vi "Configure Filter.vi"(8 "error in (no error)":errorcluster, 9 "Set Filter (1: On)":i32(ring)=1 items=["Off", "On"], 10 "Select Filter Type (0 : Frequency)":u32(ring) items=["Frequency", "Line"], 11 "VISA resource name":refnum<visa-resource-name>) -> (0 "error out":errorcluster, 3 "VISA resource name out":refnum<visa-resource-name>)   [LabVIEW 2019, in "Yokogawa WT300 Series.lvlib"]
doc: "Configures the frequency or Line filter features."
uses:
  Yokogawa WT300 Series.lvlib
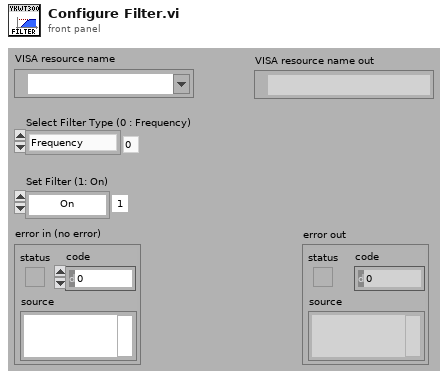
[diagram p1: front panel]
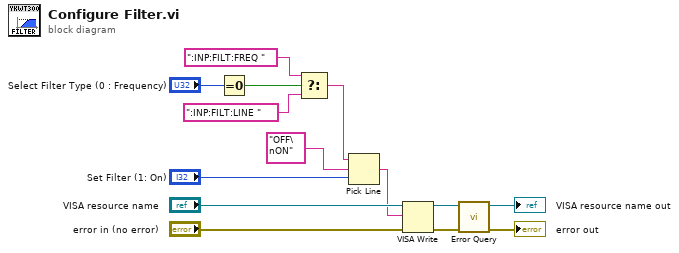
[diagram p0: block diagram]
diagram:
  n1 = Equal To 0?(x="Select Filter Type (0 : Frequency)") -> (x = 0?=w4:bool)
  n2 = Select(t=":INP:FILT:FREQ ", s=w4, f=":INP:FILT:LINE ") -> (s? t:f=w1:string)
  n3 = Pick Line ("ライン選択")(string ("")=w1, multi-line string="OFF\nON" ("複数行文字列"), line index="Set Filter (1: On)") -> (output string=w6:string)
  n4 = VISA Write ("VISA書き込み")(VISA resource name="VISA resource name", write buffer=w6, error in (no error)="error in (no error)") -> (VISA resource name out=w14:refnum<visa-resource-name>, error out=w13:errorcluster)  [unwired: 1 out]
  n5 = call "Error Query.vi"("error in (no error)"=w13, "VISA resource name"=w14) -> ("error out"=→"error out":errorcluster, "VISA resource name out"=→"VISA resource name out":refnum<visa-resource-name>)  [unwired: 6 in, 2 out]
